vi "piezoPositionToVoltage.vi"(4 "piezo":enum16{"1", "2"}(ring), 5 "mode":u16(ring) items=["um to V", "V to um"], 6 "in (array)":dbl[](array[numeric]), 7 "in":dbl) -> (2 "out (array)":dbl[](array[numeric]), 3 "out":dbl)   [LabVIEW 2017]
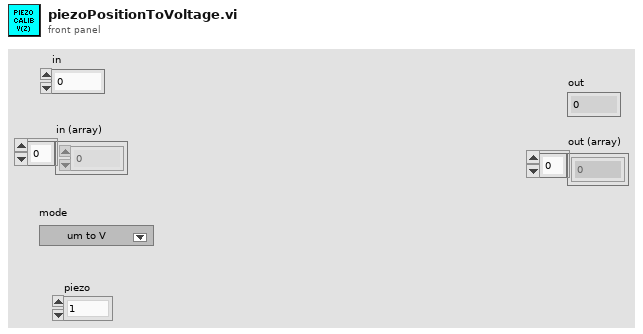
[diagram p1: front panel]
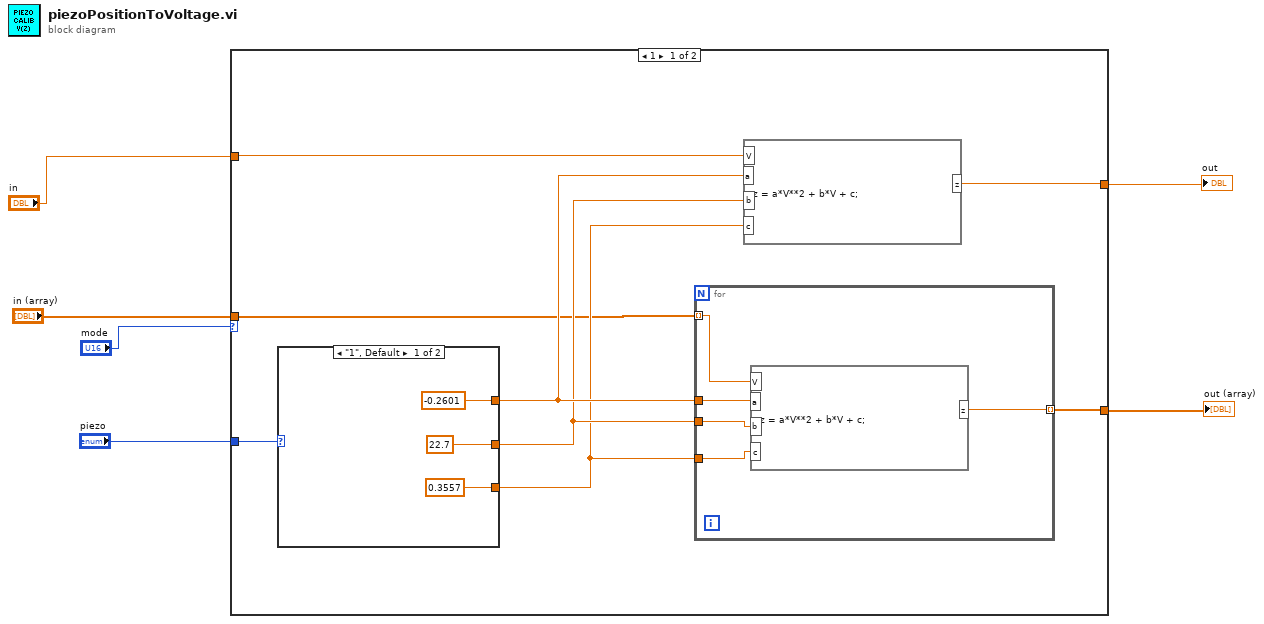
[diagram p0: block diagram]
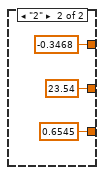
[diagram p2: hidden frame]
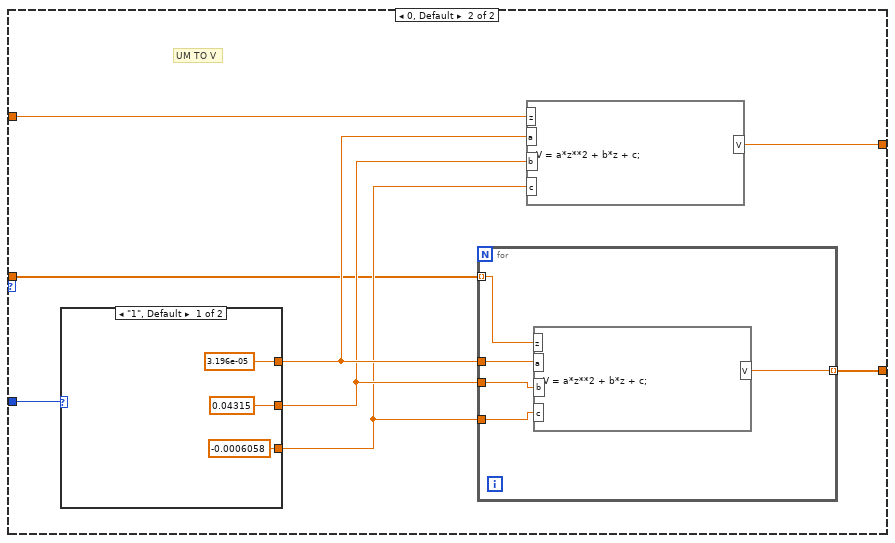
[diagram p3: hidden frame]
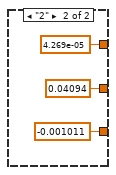
[diagram p4: hidden frame]
diagram:
  n1 = case shown="1" "mode" {
    tunnel: "piezo" -> [w9 w33]
    tunnel: "in" -> [w11 w29]
    tunnel: "in (array)" -> [w10 w28]
    tunnel: [w8 w27] -> w3
    tunnel: [w7 w26] -> w2
    frame 1 {
      n2 = case shown="\"1\", Default" w9 {
        tunnel: [-0.2601 -0.3468] -> w14
        tunnel: [22.7 23.54] -> w13
        tunnel: [0.3557 0.6545] -> w12
        frame "1", Default {
        }
        frame "2" {
        }
      }
      n3 = for {
        tunnel: w10 -> [w16] mode=indexing
        tunnel: w14 -> [w19]
        tunnel: w13 -> [w18]
        tunnel: w12 -> [w17]
        tunnel: [w15] -> w7 mode=indexing
        n4 = formula code="z = a*V**2 + b*V + c;"("a"=w19, "b"=w18, "c"=w17, "V"=w16) -> ("z"=w15:dbl)
      }
      n5 = formula code="z = a*V**2 + b*V + c;"("a"=w14, "b"=w13, "c"=w12, "V"=w11) -> ("z"=w8:dbl)
    }
    frame 0, Default {
      # "UM TO V"
      n6 = case shown="\"1\", Default" w33 {
        tunnel: [3.196e-05 4.269e-05] -> w32
        tunnel: [0.04315 0.04094] -> w31
        tunnel: [-0.0006058 -0.001011] -> w30
        frame "1", Default {
        }
        frame "2" {
        }
      }
      n7 = for {
        tunnel: w28 -> [w35] mode=indexing
        tunnel: w32 -> [w38]
        tunnel: w31 -> [w37]
        tunnel: w30 -> [w36]
        tunnel: [w34] -> w26 mode=indexing
        n8 = formula code="V = a*z**2 + b*z + c;"("a"=w38, "b"=w37, "c"=w36, "z"=w35) -> ("V"=w34:dbl)
      }
      n9 = formula code="V = a*z**2 + b*z + c;"("a"=w32, "b"=w31, "c"=w30, "z"=w29) -> ("V"=w27:dbl)
    }
  }
  "out" <- w3
  "out (array)" <- w2
